vi "LoraGroveExample.vi"() -> ()   [LabVIEW 2024]
uses:
  SubVIs/LoRaCommands.ctl
  SubVIs/Baudrates.ctl
  SubVIs/Payload.ctl
  SubVIs/Message.ctl
  SubVIs/Parameter.ctl
  SubVIs/Bandwidth.ctl
  f05726c8-305a-4e05-9821-014178edf1e9.vi
panel:
  in  "Parameter":T1={"Bandwidth"=enum."7.8kHz", "Spreading Factor (7-12)"=12, "Coding Rate (1-4)"=1, "Programmed Preamble(4-7)"=4} {"Spreading Factor (7-12)" min=7 max=12 step=1; "Coding Rate (1-4)" min=1 max=4 step=1; "Programmed Preamble(4-7)" min=4 max=7 step=1}
  out "Stopped":bool=TRUE
  in  "Stop":bool
  out "Numeric":i32
  out "Responses":string[](array[string])
  out "Response":string="+RCV=1,6,helloa,-6,11\r\n"
  in  "Read":bool
  out "Parameters":string
  out "Work Mode":string
  out "error out":errorcluster
  in  "Message":T3
  out "RF Frequency":string
  out "Identity":T4
  in  "VISA resource name":refnum<visa-resource-name>="COM15"
  in  "Payload":T5
  in  "Power":i32=1
  in  "PWD":string
  in  "Network ID":i32=1
  in  "Module Address":i32=1
  in  "Frequency":i32=868500000
  out "ModuleUID":string
  out "Version":string
  out "RF OP Power":string
  out "Network PWD":string
  out "NetworkID":string
  out "Module Address":string
  out "UART Baudrate":string
  in  "UART BaudRate":T6=enum."115200"
  in  "LoRa Command":T7=enum."Write Message"
  out "read buffer":string
  in  "Write":bool
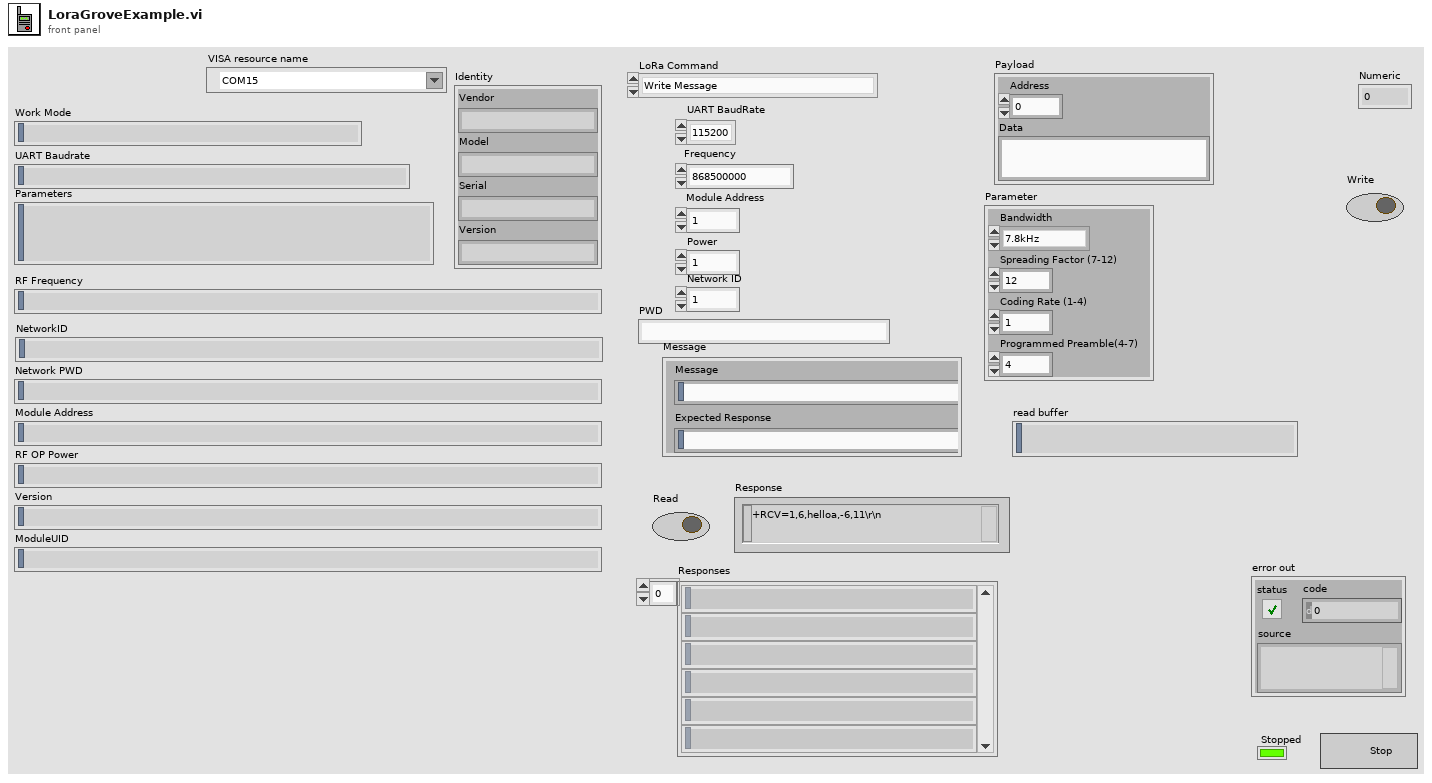
[diagram p1: front panel]
types:
  T1 = typedef "Parameter.ctl" = cluster{"Bandwidth":T2, "Spreading Factor (7-12)":u8, "Coding Rate (1-4)":u8, "Programmed Preamble(4-7)":u8}
  T2 = typedef "Bandwidth.ctl" = enum16{"125kHz", "250kHz", "500kHz", "7.8kHz", "10.4kHz", "15.6kHz", "20.8kHz", "31.25kHz", "41.7kHz", "62.5kHz"}
  T3 = typedef "Message.ctl" = cluster{"Message":string, "Expected Response":string}
  T4 = cluster{"Vendor":string, "Model":string, "Serial":string, "Version":string}
  T5 = typedef "Payload.ctl" = cluster{"Address":i32, "Data":string}
  T6 = typedef "Baudrates.ctl" = enum16{"300", "1200", "4800", "9600", "19200", "28800", "38400", "57600", "115200"}
  T7 = typedef "LoRaCommands.ctl" = enum16{"No Command - Error", "Connect", "check radio present(AT)", "Software Reset", "Set Work Mode TXRX(AT+MODE=0)", "Set Work Mode Sleep(AT+MODE=1)", "Get Work Mode(AT+MODE?)", "Set UART Baudrate", "Get UART Baudrate", "Set RF Frequency", "Get RF Frequency", "Set Module Address(AT+ADDRESS=<Addr>)", "Get Module Address(AT+ADDRESS?)", "Set Network ID(AT+NETWORKID=<ID>)", "Get Network ID(AT+NETWORKID?)", "Set Network PWD(AT+CPIN=<PW>)", "Get Network PWD(AT+CPIN?)", "Set RF OP Power(AT+CRFOP=<power>)", "Get RF OP Power(AT+CRFOP?)", "Send Data", "Receive Data", "Get Firmware Version", "Get UID of Module(AT+UID?)", "Set To Factory Defaults(AT+FACTORY)", "Set Spreading Factor", "Get Spreading Factor", "Set Bandwidth", "Get Bandwidth", "Set Coding Rate", "Get Coding Rate", "Set Preamble", "Get Preamble", "Set Active Region", "Get Active Region", "Get RF Parameters", "Set RF Parameters", "Write Message", "Disconnect"}
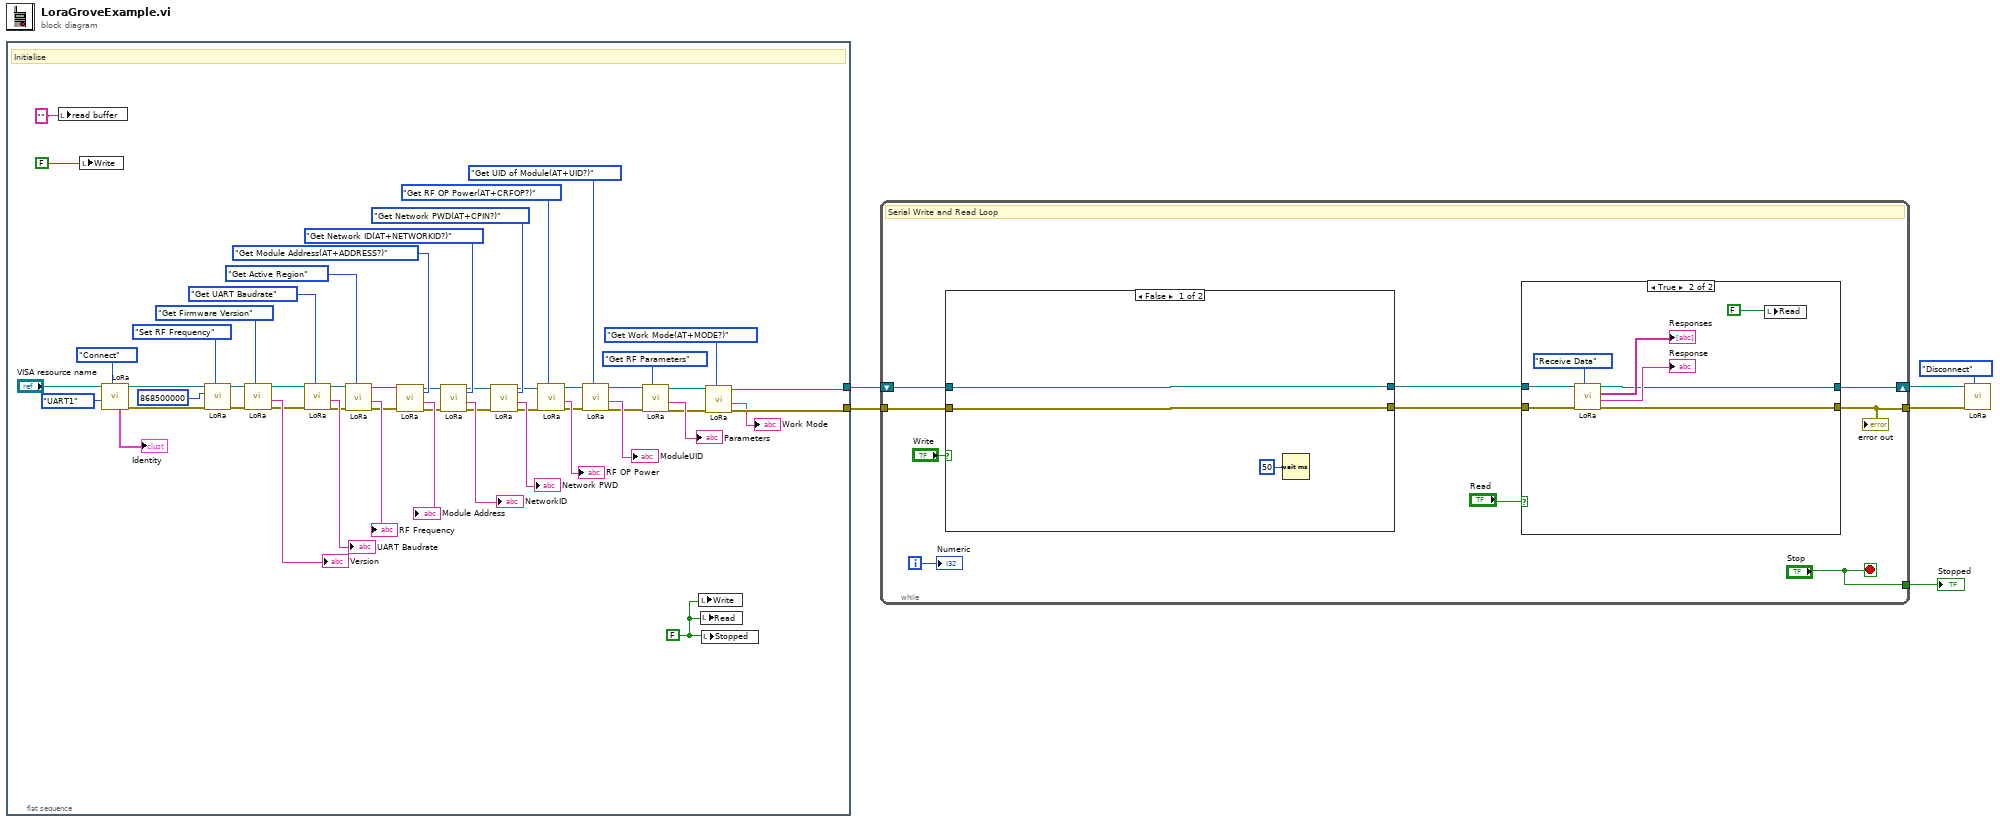
[diagram p0: block diagram]
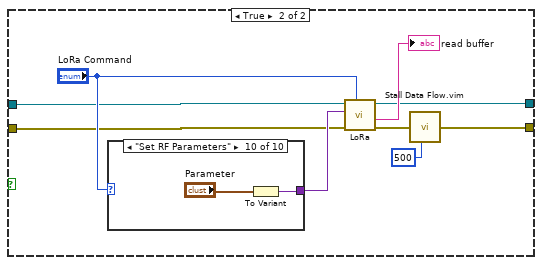
[diagram p3: hidden frame]
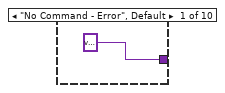
[diagram p4: hidden frame]
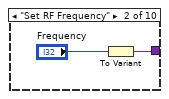
[diagram p5: hidden frame]
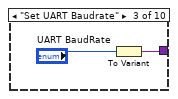
[diagram p6: hidden frame]
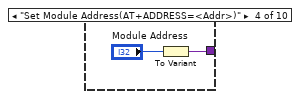
[diagram p7: hidden frame]
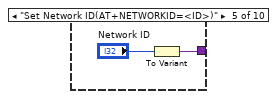
[diagram p8: hidden frame]
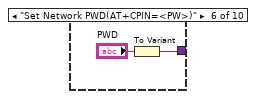
[diagram p9: hidden frame]
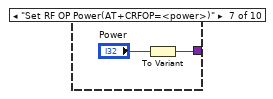
[diagram p10: hidden frame]
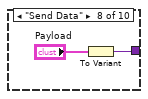
[diagram p11: hidden frame]
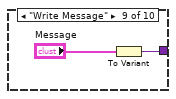
[diagram p12: hidden frame]
diagram:
  n1 = flat-sequence {
    tunnel: [w8] -> w6
    tunnel: [w9] -> w5
    frame #0 {
      w17 = FALSE ("Stopped")
      # "Initialise"
      n2 = local write "read buffer"("" ("read buffer")) -> ()
      n3 = local write "Write"(FALSE ("Read")) -> ()
      n4 = call "LoRa.vi"("LoRa Command"=LoRaCommands."Connect", "UART Connector"=enum16{"UART0", "UART1"}."UART1", "VISA resource name"="VISA resource name") -> ("error out"=w20:errorcluster, "VISA resource name out"=w21:refnum<visa-resource-name>, "Identity"=→"Identity":T4)  [unwired: 4 in, 2 out]
      n5 = call "LoRa.vi"("LoRa Command"=LoRaCommands."Set RF Frequency", "error in (no error)"=w20, "Variant"=868500000 ("Frequency"), "VISA resource name"=w21) -> ("error out"=w18:errorcluster, "VISA resource name out"=w19:refnum<visa-resource-name>)  [unwired: 3 in, 3 out]
      n6 = call "LoRa.vi"("LoRa Command"=LoRaCommands."Get Firmware Version", "error in (no error)"=w18, "VISA resource name"=w19) -> ("error out"=w48:errorcluster, "read buffer"=→"Version":string, "VISA resource name out"=w49:refnum<visa-resource-name>)  [unwired: 4 in, 2 out]
      n7 = call "LoRa.vi"("LoRa Command"=LoRaCommands."Get UART Baudrate", "error in (no error)"=w48, "VISA resource name"=w49) -> ("error out"=w44:errorcluster, "read buffer"=→"UART Baudrate":string, "VISA resource name out"=w45:refnum<visa-resource-name>)  [unwired: 4 in, 2 out]
      n8 = call "LoRa.vi"("LoRa Command"=LoRaCommands."Get Active Region", "error in (no error)"=w44, "VISA resource name"=w45) -> ("error out"=w40:errorcluster, "read buffer"=→"RF Frequency":string, "VISA resource name out"=w41:refnum<visa-resource-name>)  [unwired: 4 in, 2 out]
      n9 = call "LoRa.vi"("LoRa Command"=LoRaCommands."Get Module Address(AT+ADDRESS?)", "error in (no error)"=w40, "VISA resource name"=w41) -> ("error out"=w36:errorcluster, "read buffer"=→"Module Address":string, "VISA resource name out"=w37:refnum<visa-resource-name>)  [unwired: 4 in, 2 out]
      n10 = call "LoRa.vi"("LoRa Command"=LoRaCommands."Get Network ID(AT+NETWORKID?)", "error in (no error)"=w36, "VISA resource name"=w37) -> ("error out"=w32:errorcluster, "read buffer"=→"NetworkID":string, "VISA resource name out"=w33:refnum<visa-resource-name>)  [unwired: 4 in, 2 out]
      n11 = call "LoRa.vi"("LoRa Command"=LoRaCommands."Get Network PWD(AT+CPIN?)", "error in (no error)"=w32, "VISA resource name"=w33) -> ("error out"=w27:errorcluster, "read buffer"=→"Network PWD":string, "VISA resource name out"=w26:refnum<visa-resource-name>)  [unwired: 4 in, 2 out]
      n12 = call "LoRa.vi"("LoRa Command"=LoRaCommands."Get RF OP Power(AT+CRFOP?)", "error in (no error)"=w27, "VISA resource name"=w26) -> ("error out"=w24:errorcluster, "read buffer"=→"RF OP Power":string, "VISA resource name out"=w25:refnum<visa-resource-name>)  [unwired: 4 in, 2 out]
      n13 = call "LoRa.vi"("LoRa Command"=LoRaCommands."Get UID of Module(AT+UID?)", "error in (no error)"=w24, "VISA resource name"=w25) -> ("error out"=w15:errorcluster, "read buffer"=→"ModuleUID":string, "VISA resource name out"=w16:refnum<visa-resource-name>)  [unwired: 4 in, 2 out]
      n14 = call "LoRa.vi"("LoRa Command"=LoRaCommands."Get RF Parameters", "error in (no error)"=w15, "VISA resource name"=w16) -> ("error out"=w11:errorcluster, "read buffer"=→"Parameters":string, "VISA resource name out"=w12:refnum<visa-resource-name>)  [unwired: 4 in, 2 out]
      n15 = local write "Write"(w17) -> ()
      n16 = local write "Read"(w17) -> ()
      n17 = local write "Stopped"(w17) -> ()
      n18 = call "LoRa.vi"("LoRa Command"=LoRaCommands."Get Work Mode(AT+MODE?)", "error in (no error)"=w11, "VISA resource name"=w12) -> ("error out"=w9:errorcluster, "read buffer"=→"Work Mode":string, "VISA resource name out"=w8:refnum<visa-resource-name>)  [unwired: 4 in, 2 out]
    }
  }
  n19 = while {
    shift-right: [w61] -> w2
    shift-left: w6 -> [w69]
    tunnel: w5 -> [w68]
    tunnel: [w62] -> w3
    tunnel: ["Stop"] -> w1
    i -> [w66]
    stop <- "Stop" stop-if-true
    # "Serial Write and Read Loop"
    n20 = case shown="False" "Write" {
      tunnel: w69 -> [w82 w88]
      tunnel: w68 -> [w81 w87]
      tunnel: [w82 w86] -> w64
      tunnel: [w81 w84] -> w63
      frame False {
        n21 = Wait (ms)(milliseconds to wait=u32 50) -> ()  [unwired: 1 out]
      }
      frame True {
        n22 = case shown="\"Set RF Parameters\"" "LoRa Command" {
          tunnel: [variant ("Variant") w94 w96 w98 w100 w102 w104 w106 w108 w110] -> w89
          frame "No Command - Error", Default {
          }
          frame "Set RF Frequency" {
            n23 = To Variant(anything="Frequency") -> (Variant=w94:variant)
          }
          frame "Set UART Baudrate" {
            n24 = To Variant(anything="UART BaudRate") -> (Variant=w96:variant)
          }
          frame "Set Module Address(AT+ADDRESS=<Addr>)" {
            n25 = To Variant(anything="Module Address") -> (Variant=w98:variant)
          }
          frame "Set Network ID(AT+NETWORKID=<ID>)" {
            n26 = To Variant(anything="Network ID") -> (Variant=w100:variant)
          }
          frame "Set Network PWD(AT+CPIN=<PW>)" {
            n27 = To Variant(anything="PWD") -> (Variant=w102:variant)
          }
          frame "Set RF OP Power(AT+CRFOP=<power>)" {
            n28 = To Variant(anything="Power") -> (Variant=w104:variant)
          }
          frame "Send Data" {
            n29 = To Variant(anything="Payload") -> (Variant=w106:variant)
          }
          frame "Write Message" {
            n30 = To Variant(anything="Message") -> (Variant=w108:variant)
          }
          frame "Set RF Parameters" {
            n31 = To Variant(anything="Parameter") -> (Variant=w110:variant)
          }
        }
        n32 = call "LoRa.vi"("LoRa Command"="LoRa Command", "error in (no error)"=w87, "Variant"=w89, "VISA resource name"=w88) -> ("error out"=w85:errorcluster, "read buffer"=→"read buffer":string, "VISA resource name out"=w86:refnum<visa-resource-name>)  [unwired: 3 in, 2 out]
        n33 = call "Stall Data Flow.vim"("value in"=w85, "milliseconds to wait"=u32 500) -> ("value out"=w84:errorcluster)  [unwired: 1 out]
      }
    }
    n34 = case shown="True" "Read" {
      tunnel: w64 -> [w71 w79]
      tunnel: w63 -> [w70 w78]
      tunnel: [w70 w75] -> w62
      tunnel: [w71 w74] -> w61
      frame False {
      }
      frame True {
        n35 = call "LoRa.vi"("LoRa Command"=LoRaCommands."Receive Data", "error in (no error)"=w78, "VISA resource name"=w79) -> ("error out"=w75:errorcluster, "read buffer"=→"Response":string, "Returned Data"=→"Responses":string[], "VISA resource name out"=w74:refnum<visa-resource-name>)  [unwired: 4 in, 1 out]
        n36 = local write "Read"(FALSE) -> ()
      }
    }
    "error out" <- w62
    "Numeric" <- w66
  }
  "Stopped" <- w1
  n37 = call "LoRa.vi"("LoRa Command"=LoRaCommands."Disconnect", "error in (no error)"=w3, "VISA resource name"=w2) -> ()  [unwired: 4 in, 5 out]
